vi "catch2.vi"(11 "NXT/EV3":T1) -> (3 "NXT/EV3 2":T1)   [LabVIEW 2016]
uses:
  <vilib>/NXT/Subs/LVHSConnector.ctl
  <vilib>/NXT/LegoClasses/BrickReference/BrickReference.lvclass
  <vilib>/NXT/Block Support/NXT_OutputPort.ctl
  <vilib>/NXT/NXTIO Xnodes/NXTIONodeSubVIs/NXTMoveMotors.vi
  <vilib>/NXT/Dual Mode Library/Waits/Wait_Rotation.vi
  <vilib>/NXT/NXTIO Xnodes/NXTIONodeSubVIs/NXTStopMotors.vi
  <vilib>/NXT/Dual Mode Library/Waits/Wait_Num.vi
  <vilib>/NXT/NXTIO Xnodes/AddressXNode/NXTIOAddress.xnode
  <vilib>/NXT/NXTIO Xnodes/NXTIOXNode/NXTIO.xnode
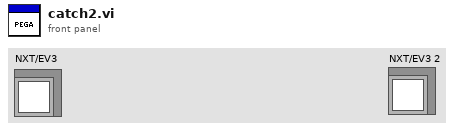
[diagram p1: front panel]
types:
  T1 = typedef "LVHSConnector.ctl" = refnum<class "BrickReference.lvclass">
  T2 = typedef "NXT_OutputPort.ctl" = u8
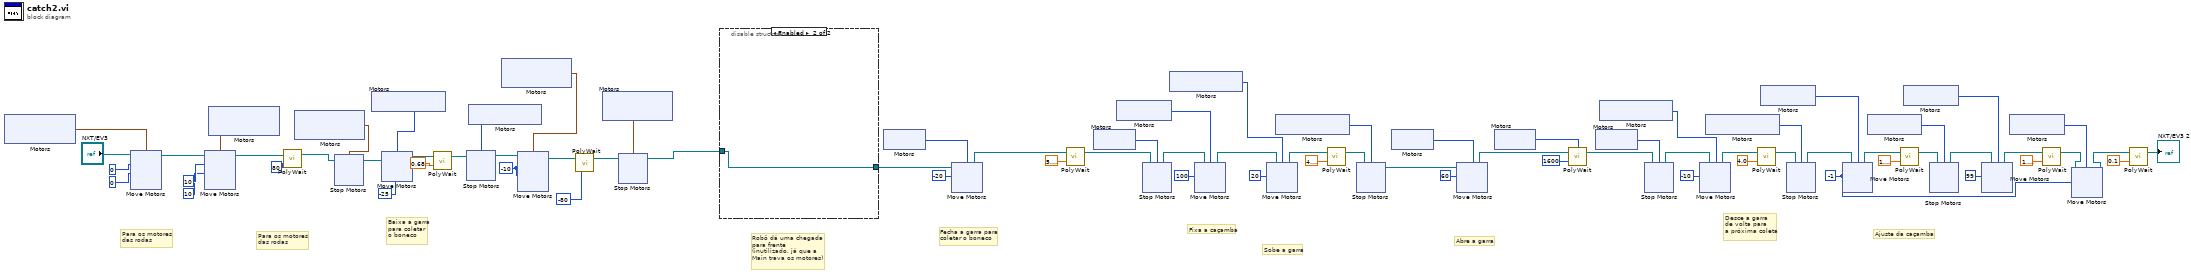
[diagram p0: block diagram]
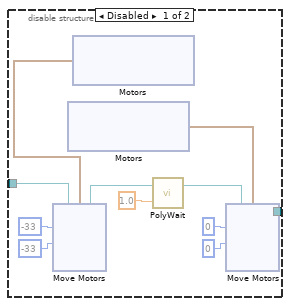
[diagram p2: hidden frame]
diagram:
  w13 = i8 -10 ("Power/Speed 1")
  w23 = i8 -1 ("Power/Speed 1")
  # "Para os motores\ndas rodas"
  # "Ajuste da caçamba"
  # "Desce a garra\nde volta para\na próxima coleta"
  # "Abre a garra"
  # "Sobe a garra"
  # "Fixa a caçamba"
  # "Fecha a garra para\ncoletar o boneco"
  # "Robô dá uma chegada\npara frente\n(inutilizado, já que a \nMain trava os motores)"
  # "Baixa a garra\npara coletar\no boneco"
  # "Para os motores\ndas rodas"
  n1 = xnode "Motors"() -> ("Motor"=w34:cluster{"Port":T2, "Port":T2})
  n2 = xnode "Move Motors"("Power/Speed 2"=i8 0 ("Power/Speed 1"), "Power/Speed 1"=i8 0, "Motors"=w34, "NXT/EV3"="NXT/EV3") -> ("NXT/EV3"=w21:T1)
  n3 = xnode "Motors"() -> ("Motor"=w22:cluster{"Port":T2, "Port":T2})
  n4 = xnode "Move Motors"("Power/Speed 2"=i8 10 ("Power/Speed 1"), "Power/Speed 1"=i8 10, "Motors"=w22, "NXT/EV3"=w21) -> ("NXT/EV3"=w18:T1)
  n5 = call-poly <vilib>:"PolyWait.vi"("Position Change (180)"=80, "NXT/EV3"=w18) -> ("NXT/EV3"=w11:T1)  [unwired: 2 in]
  n6 = xnode "Motors"() -> ("Motor"=w10:cluster{"Port":T2, "Port":T2})
  n7 = xnode "Stop Motors"("Motors"=w10, "NXT/EV3"=w11) -> ("NXT/EV3"=w15:T1)
  n8 = xnode "Motors"() -> ("Motor"=w8:T2)
  n9 = xnode "Move Motors"("Power/Speed 1"=i8 -25, "Motors"=w8, "NXT/EV3"=w15) -> ("NXT/EV3"=w5:T1)
  n10 = call-poly <vilib>:"PolyWait.vi"("Time (1 sec)"=sgl 0.69, "NXT/EV3"=w5) -> ("NXT/EV3"=w4:T1)  [unwired: 2 in]
  n11 = xnode "Motors"() -> ("Motor"=w7:T2)
  n12 = xnode "Stop Motors"("Motors"=w7, "NXT/EV3"=w4) -> ("NXT/EV3"=w9:T1)
  n13 = xnode "Motors"() -> ("Motor"=w14:cluster{"Port":T2, "Port":T2})
  n14 = xnode "Move Motors"("Power/Speed 2"=w13, "Power/Speed 1"=w13, "Motors"=w14, "NXT/EV3"=w9) -> ("NXT/EV3"=w12:T1)
  n15 = call-poly <vilib>:"PolyWait.vi"("Position Change (180)"=-80, "NXT/EV3"=w12) -> ("NXT/EV3"=w3:T1)  [unwired: 2 in]
  n16 = xnode "Motors"() -> ("Motor"=w1:cluster{"Port":T2, "Port":T2})
  n17 = xnode "Stop Motors"("Motors"=w1, "NXT/EV3"=w3) -> ("NXT/EV3"=w2:T1)
  n18 = disable-structure shown="Enabled" {
    disable-tunnel: w2 -> [w85 w106]
    disable-tunnel: [w79 w106] -> w31
    frame Disabled {
      n19 = xnode "Motors"() -> ("Motor"=w87:cluster{"Port":T2, "Port":T2})
      n20 = xnode "Motors"() -> ("Motor"=w86:cluster{"Port":T2, "Port":T2})
      n21 = xnode "Move Motors"("Power/Speed 2"=i8 -33, "Power/Speed 1"=i8 -33, "Motors"=w86, "NXT/EV3"=w85) -> ("NXT/EV3"=w82:T1)
      n22 = call-poly <vilib>:"PolyWait.vi"("Time (1 sec)"=sgl 1.0, "NXT/EV3"=w82) -> ("NXT/EV3"=w80:T1)  [unwired: 2 in]
      n23 = xnode "Move Motors"("Power/Speed 2"=i8 0, "Power/Speed 1"=i8 0, "Motors"=w87, "NXT/EV3"=w80) -> ("NXT/EV3"=w79:T1)
    }
    frame Enabled {
    }
  }
  n24 = xnode "Motors"() -> ("Motor"=w62:T2)
  n25 = xnode "Move Motors"("Power/Speed 1"=i8 -20, "Motors"=w62, "NXT/EV3"=w31) -> ("NXT/EV3"=w60:T1)
  n26 = call-poly <vilib>:"PolyWait.vi"("Time (1 sec)"=sgl 5.1, "NXT/EV3"=w60) -> ("NXT/EV3"=w58:T1)  [unwired: 2 in]
  n27 = xnode "Motors"() -> ("Motor"=w59:T2)
  n28 = xnode "Motors"() -> ("Motor"=w50:T2)
  n29 = xnode "Stop Motors"("Motors"=w59, "NXT/EV3"=w58) -> ("NXT/EV3"=w44:T1)
  n30 = xnode "Motors"() -> ("Motor"=w69:T2)
  n31 = xnode "Move Motors"("Power/Speed 1"=i8 100, "Motors"=w50, "NXT/EV3"=w44) -> ("NXT/EV3"=w43:T1)
  n32 = xnode "Move Motors"("Power/Speed 1"=i8 20, "Motors"=w69, "NXT/EV3"=w43) -> ("NXT/EV3"=w73:T1)
  n33 = xnode "Motors"() -> ("Motor"=w70:T2)
  n34 = call-poly <vilib>:"PolyWait.vi"("Time (1 sec)"=sgl 4.7, "NXT/EV3"=w73) -> ("NXT/EV3"=w71:T1)  [unwired: 2 in]
  n35 = xnode "Stop Motors"("Motors"=w70, "NXT/EV3"=w71) -> ("NXT/EV3"=w56:T1)
  n36 = xnode "Motors"() -> ("Motor"=w57:T2)
  n37 = xnode "Move Motors"("Power/Speed 1"=i8 60, "Motors"=w57, "NXT/EV3"=w56) -> ("NXT/EV3"=w54:T1)
  n38 = xnode "Motors"() -> ("Motor"=w27:T2)
  n39 = call-poly <vilib>:"PolyWait.vi"("Position Change (180)"=1600, "NXT/EV3"=w54, "Port (Port A)"=w27) -> ("NXT/EV3"=w53:T1)  [unwired: 1 in]
  n40 = xnode "Motors"() -> ("Motor"=w42:T2)
  n41 = xnode "Motors"() -> ("Motor"=w51:T2)
  n42 = xnode "Stop Motors"("Motors"=w42, "NXT/EV3"=w53) -> ("NXT/EV3"=w52:T1)
  n43 = xnode "Move Motors"("Power/Speed 1"=i8 -10, "Motors"=w51, "NXT/EV3"=w52) -> ("NXT/EV3"=w66:T1)
  n44 = xnode "Motors"() -> ("Motor"=w63:T2)
  n45 = call-poly <vilib>:"PolyWait.vi"("Time (1 sec)"=sgl 4.0, "NXT/EV3"=w66) -> ("NXT/EV3"=w64:T1)  [unwired: 2 in]
  n46 = xnode "Motors"() -> ("Motor"=w41:T2)
  n47 = xnode "Stop Motors"("Motors"=w63, "NXT/EV3"=w64) -> ("NXT/EV3"=w40:T1)
  n48 = xnode "Move Motors"("Power/Speed 1"=w23, "Motors"=w41, "NXT/EV3"=w40) -> ("NXT/EV3"=w38:T1)
  n49 = xnode "Motors"() -> ("Motor"=w37:T2)
  n50 = call-poly <vilib>:"PolyWait.vi"("Time (1 sec)"=sgl 1.3, "NXT/EV3"=w38) -> ("NXT/EV3"=w36:T1)  [unwired: 2 in]
  n51 = xnode "Motors"() -> ("Motor"=w48:T2)
  n52 = xnode "Stop Motors"("Motors"=w37, "NXT/EV3"=w36) -> ("NXT/EV3"=w35:T1)
  n53 = xnode "Move Motors"("Power/Speed 1"=i8 99, "Motors"=w48, "NXT/EV3"=w35) -> ("NXT/EV3"=w46:T1)
  n54 = xnode "Motors"() -> ("Motor"=w26:T2)
  n55 = call-poly <vilib>:"PolyWait.vi"("Time (1 sec)"=sgl 1.3, "NXT/EV3"=w46) -> ("NXT/EV3"=w25:T1)  [unwired: 2 in]
  n56 = xnode "Move Motors"("Power/Speed 1"=w23, "Motors"=w26, "NXT/EV3"=w25) -> ("NXT/EV3"=w24:T1)
  n57 = call-poly <vilib>:"PolyWait.vi"("Time (1 sec)"=0.1, "NXT/EV3"=w24) -> ("NXT/EV3"=→"NXT/EV3 2":T1)  [unwired: 2 in]
